vi "ReadingMatFile.vi"() -> ()   [LabVIEW 2015]
panel:
  in  "stop":bool
  out "Y":dbl
  out "X":dbl
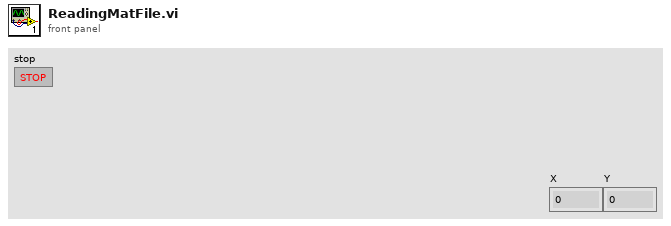
[diagram p1: front panel]
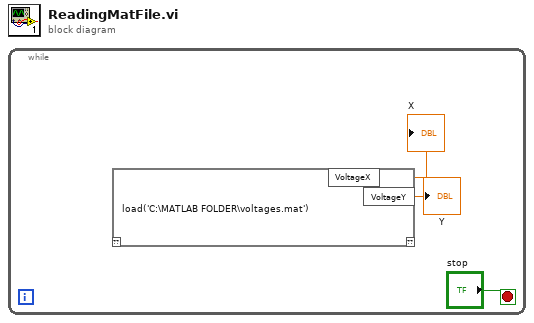
[diagram p0: block diagram]
diagram:
  n1 = while {
    stop <- "stop" stop-if-true
    n2 = script code="load('C:\\MATLAB FOLDER\\voltages.mat')"() -> ("VoltageX"=→"X":dbl, "VoltageY"=→"Y":dbl)  [unwired: 1 in, 1 out]
  }
